vi "Write trigger type (Edge).vi"(8 "error in (no error)":errorcluster, 10 "trigger type (Edge)":i32(ring)=1 items=["Edge"=1, "TV"=5, "Runt"=3, "Glitch"=4, "Width"=2, "AC Line"=7, "Immediate"=6], 11 "Configure Trigger Msg in":refnum<class "Configure Trigger Msg.lvclass">) -> (0 "error out":errorcluster, 3 "Configure Trigger Msg out":refnum<class "Configure Trigger Msg.lvclass">)   [LabVIEW 2015, in "CS++Scope.lvlib" / "Configure Trigger Msg.lvclass"]
uses:
  Configure Trigger Msg.lvclass
  Configure Trigger Msg.lvclass/Configure Trigger Msg.ctl
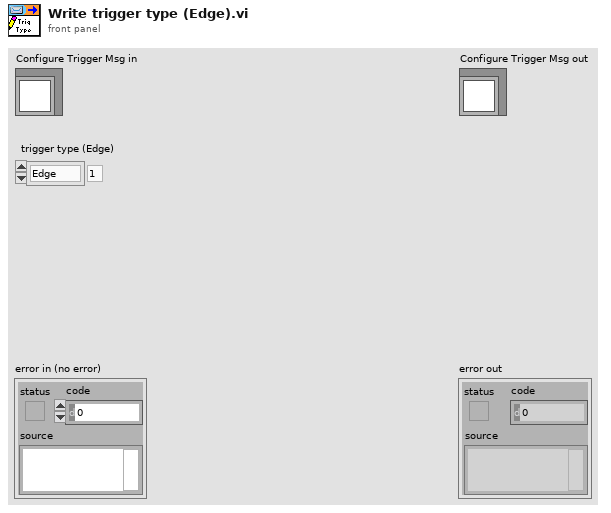
[diagram p1: front panel]
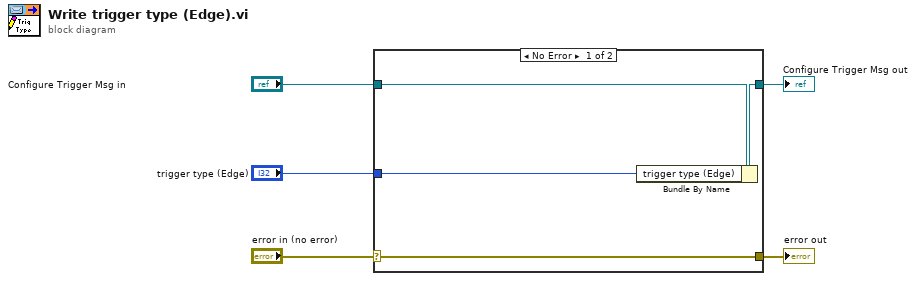
[diagram p0: block diagram]
diagram:
  n1 = case shown="No Error" "error in (no error)" {
    selector: "error in (no error)" -> [w9 w10]
    tunnel: [w9 w10] -> w4
    tunnel: [w7 w11] -> w2
    tunnel: "Configure Trigger Msg in" -> [w8 w11]
    tunnel: "trigger type (Edge)" -> [w6 _]
    frame No Error {
      n2 = Bundle By Name(cluster=w8, "trigger type (Edge)"=w6) -> (w7:refnum<class "Configure Trigger Msg.lvclass">)
    }
    frame Error {
    }
  }
  "error out" <- w4
  "Configure Trigger Msg out" <- w2
